vi "Get Result.vi"(8 "error in (no error)":errorcluster, 11 "Red Pitaya Lock-in Driver in":refnum<class "Red Pitaya Lock-in Driver.lvclass">) -> (0 "error out":errorcluster, 2 "Result":refnum<class "Acquired Result.lvclass">, 3 "Red Pitaya Lock-in Driver out":refnum<class "Red Pitaya Lock-in Driver.lvclass">)   [LabVIEW 2019, in "Red Pitaya Lock-in Driver.lvclass"]
uses:
  Red Pitaya Lock-in Driver.lvclass
  C:/GitHub/NHMFL_Core/Libraries/Instruments/Instrument Driver/Lock-in Driver/Lock-in Driver.lvclass
  C:/GitHub/NHMFL_Core/Libraries/Instruments/Instrument Driver/Instrument Driver.lvclass
  Instruments/Results/Acquired Result/Acquired Result.lvclass
  Red Pitaya Lock-in Driver.lvclass/Red Pitaya Lock-in Driver.ctl
  Read RP Instrument.vi
  Instruments/Instrument Driver/Read Recorder name.vi
  Write RP Instrument.vi
  Instruments/Instrument Driver/Lock-in Driver/Read Lock-in configuration.vi
  RP Instrument/RP Instrument.lvclass
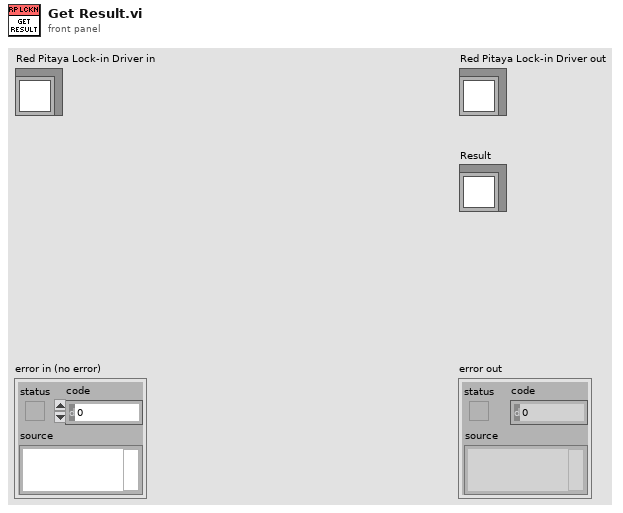
[diagram p1: front panel]
types:
  T1 = typedef "Lock-in Configuration.ctl" = cluster{"Frequency":dbl, "Time constant":dbl, "Synchronous":bool, "Channels":i32[]}
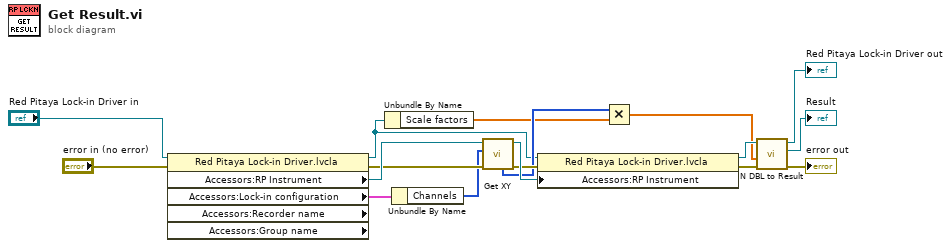
[diagram p0: block diagram]
diagram:
  n1 = property class="Red Pitaya Lock-in Driver.lvcla" props=["Accessors:RP Instrument", "Accessors:Lock-in configuration", "Accessors:Recorder name", "Accessors:Group name"](reference="Red Pitaya Lock-in Driver in", error in="error in (no error)") -> (reference out=w2:refnum<class "Red Pitaya Lock-in Driver.lvclass">, error out=w13:errorcluster, "Accessors:RP Instrument"=w16:refnum<class "RP Instrument.lvclass">, "Accessors:Lock-in configuration"=w11:T1)  [unwired: 2 out]
  n2 = Unbundle By Name(w2) -> ("Scale factors"=w1:dbl[])
  n3 = Unbundle By Name(w11) -> ("Channels"=w9:i32[])
  n4 = call-dynamic "Get XY.vi"("error in (no error)"=w13, "Channels"=w9, "RP Instrument in"=w16) -> ("error out"=w12:errorcluster, "RP Instrument out"=w15:refnum<class "RP Instrument.lvclass">, "Signal"=w10:i32[])  [unwired: 6 in]
  n5 = property class="Red Pitaya Lock-in Driver.lvcla"(reference=w2, error in=w12, "Accessors:RP Instrument"=w15) -> (reference out=w8:refnum<class "Red Pitaya Lock-in Driver.lvclass">, error out=w4:errorcluster)
  n6 = Multiply(x=w10, y=w1) -> (x*y=w5:dbl[])
  n7 = call-dynamic "N DBL to Result.vi"("error in (no error)"=w4, "Data"=w5, "Instrument Driver in"=w8) -> ("error out"=→"error out":errorcluster, "Result out"=→"Result":refnum<class "Acquired Result.lvclass">, "Instrument Driver out"=→"Red Pitaya Lock-in Driver out":refnum<class "Red Pitaya Lock-in Driver.lvclass">)  [unwired: 6 in]
